vi "sub_getQueueSizes.vi"(11 "queues":T1) -> (3 "output cluster":cluster{"q1":i32, "q2":i32, "q3":i32})   [LabVIEW 2018]
uses:
  guess.ctl
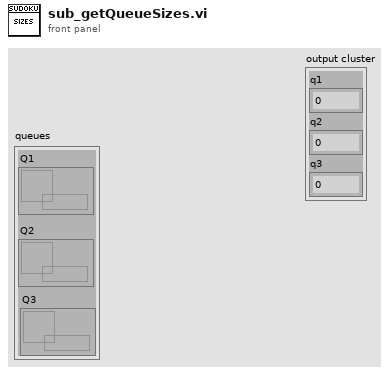
[diagram p1: front panel]
types:
  T1 = cluster{"Q1":refnum<queue>, "Q2":refnum<queue>, "Q3":refnum<queue>}
  T2 = cluster{"# elements in queue":i32, "# elements in queue":i32, "# elements in queue":i32}
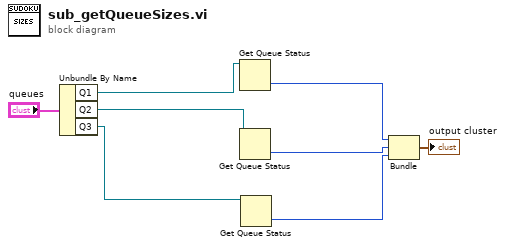
[diagram p0: block diagram]
diagram:
  n1 = Unbundle By Name("queues") -> ("Q1"=w7:refnum<queue>, "Q2"=w6:refnum<queue>, "Q3"=w5:refnum<queue>)
  n2 = Get Queue Status(queue=w7) -> (# elements in queue=w4:i32)  [unwired: 2 in, 7 out]
  n3 = Get Queue Status(queue=w6) -> (# elements in queue=w3:i32)  [unwired: 2 in, 7 out]
  n4 = Get Queue Status(queue=w5) -> (# elements in queue=w2:i32)  [unwired: 2 in, 7 out]
  n5 = Bundle("# elements in queue"=w4, "# elements in queue"=w3, "# elements in queue"=w2) -> (→"output cluster":T2)  [unwired: 1 in]
